vi "5.4-4.7.4-How Client.vi"() -> ()   [LabVIEW 2010]
doc: "This VI implements a client for the Named Service UDP Server.vi.\nIt connects to a service by specifying the server address and the name of the service. After sending a 'Hello' string to the server, the client receives the string sent by the server, displays the string and closes the connection.\n\n<b>Note:</b> This VI is built to work with the Named Service UDP Server.vi in UDP.llb."
uses:
  4-High Neurons/4.4-How Sensor Typedef.ctl
  4-High Neurons/4.0-Midbrain State.ctl
  4-High Neurons/4.0-Timing Badass.ctl
  <vilib>/Utility/tcp.llb/UDP Multicast Open.vi
  5.0-Global.vi
  5.7-UDP/5.7-UDP Check Checksum.vi
  <vilib>/addons/internet/NI_InternetTK_Common_VIs.lvlib
panel:
  out "Super Heart Beat":T1
  out "data":T2
  out "Error":errorcluster
  in  "stop":bool
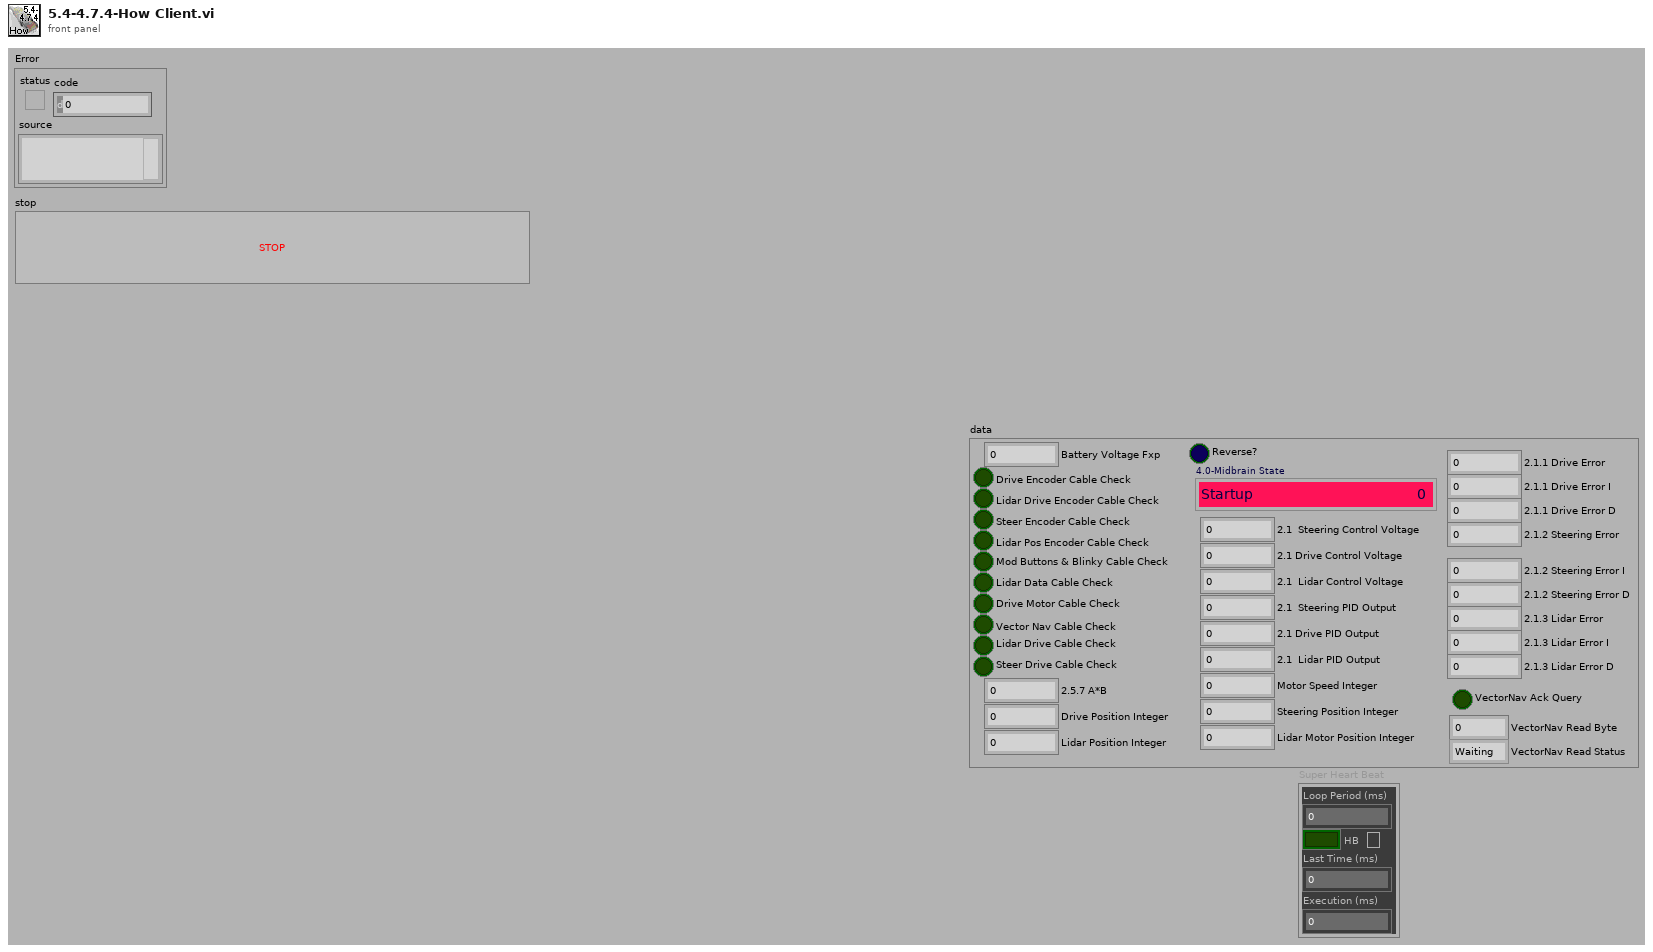
[diagram p1: front panel]
types:
  T1 = typedef "4.0-Timing Badass.ctl" = cluster{"Loop Period (ms)":u32, "HB":bool, "Last Time (ms)":u32, "Execution (ms)":u32}
  T2 = typedef "4.4-How Sensor Typedef.ctl" = cluster{"Motor Speed Integer":i32, "Drive Position Integer":i32, "Lidar Position Integer":i32, "Lidar Motor Position Integer":i32, "Steering Position Integer":i32, "Battery Voltage Fxp":dbl, "Drive Encoder Cable Check":bool, "Lidar Drive Encoder Cable Check":bool, "Steer Encoder Cable Check":bool, "Lidar Pos Encoder Cable Check":bool, "Mod Buttons & Blinky Cable Check":bool, "Lidar Data Cable Check":bool, "Drive Motor Cable Check":bool, "Vector Nav Cable Check":bool, "Lidar Drive Cable Check":bool, "Steer Drive Cable Check":bool, "Reverse?":bool, "2.1  Steering Control Voltage":dbl, "2.1 Drive Control Voltage":dbl, "2.1  Lidar Control Voltage":dbl, "2.5.7 A*B":dbl, "2.1  Steering PID Output":dbl, "2.1 Drive PID Output":dbl, "2.1  Lidar PID Output":dbl, "2.1.1 Drive Error":dbl, "2.1.1 Drive Error I":dbl, "2.1.1 Drive Error D":dbl, "2.1.2 Steering Error":dbl, "2.1.2 Steering Error I":dbl, "2.1.2 Steering Error D":dbl, "2.1.3 Lidar Error":dbl, "2.1.3 Lidar Error I":dbl, "2.1.3 Lidar Error D":dbl, "VectorNav Ack Query":bool, "VectorNav Read Byte":u8, "VectorNav Read Status":enum16{"Waiting", "Reading", "Done"}, "4.0-Midbrain State":T3}
  T3 = typedef "4.0-Midbrain State.ctl" = enum16{"Startup", "Waiting to Run", "Running-OlinOval", "Running-ChannelFollow", "Running-WallFollow", "Running-OpenTransit", "Running-Joystick Training", "Shutdown", "Restart"}
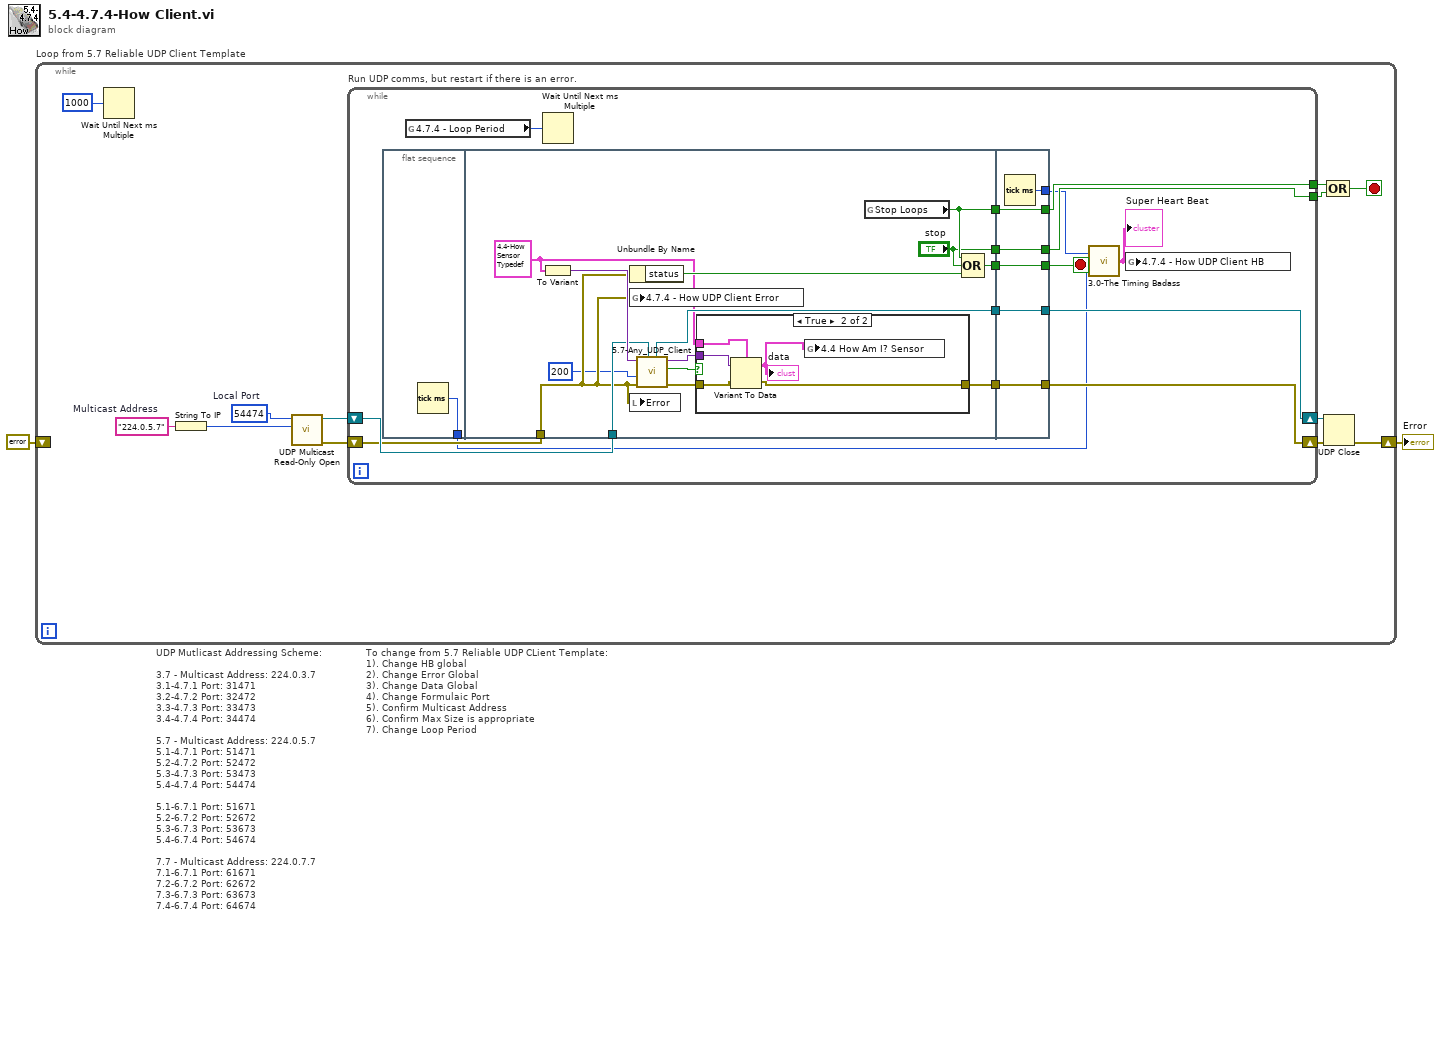
[diagram p0: block diagram]
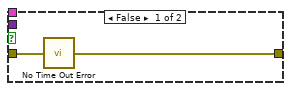
[diagram p2: hidden frame]
diagram:
  # "To change from 5.7 Reliable UDP CLient Template:\n1). Change HB global\n2). Change Error Global\n3). Change Data Global\n4). Change Formulaic Port\n5). Confirm Multicast Address\n6). Confirm Max Size is appropriate\n7). Change Loop Period"
  # "UDP Mutlicast Addressing Scheme:\n\n3.7 - Multicast Address: 224.0.3.7\n3.1-4.7.1 Port: 31471\n3.2-4.7.2 Port: 32472\n3.3-4.7.3 Port: 33473\n3.4-4.7.4 Port: 34474\n\n5.7 - Multicast Address: 224.0.5.7\n5.1-4.7.1 Port: 51471\n5.2-4.7.2 Port: 52472\n5.3-4.7.3 Port: 53473\n5.4-4.7.4 Port: 54474\n\n5.1-6.7.1 Port: 51671\n5.2-6.7.2 Port: 52672\n5.3-6.7.3 Port: 53673\n5.4-6.7.4 Port: 54674\n\n7.7 - Multicast Address: 224.0.7.7\n7.1-6.7.1 Port: 61671\n7.2-6.7.2 Port: 62672\n7.3-6.7.3 Port: 63673\n7.4-6.7.4 Port: 64674"
  n1 = while "Loop from 5.7 Reliable UDP Client Template" {
    shift-right: [w9] -> w2
    shift-left: errorcluster {"status"=FALSE, "code"=0, "source"=""} ("error out") -> [_]
    stop <- w12 stop-if-true
    w5 = u16 54474  # Local Port
    w7 = "224.0.5.7"  # Multicast Address
    n2 = Wait Until Next ms Multiple(millisecond multiple=u32 1000) -> ()  [unwired: 1 out]
    n3 = String To IP(1:w7) -> (0:w6:u32)
    n4 = call-poly <vilib>:"UDP Multicast Read-Only Open.vi"("multicast addr"=w6, "port"=w5) -> ("error out"=w3:errorcluster, "connection ID"=w4:refnum<k16>)  [unwired: 2 in, 6 out]
    n5 = while "Run UDP comms, but restart if there is an error." {
      tunnel: [w29] -> w14
      tunnel: [w28] -> w13
      shift-right: [w26] -> w11
      shift-left: w4 -> [w27]
      shift-right: [w25] -> w10
      shift-left: w3 -> [w24]
      stop <- w30 stop-if-true
      n6 = flat-sequence {
        tunnel: [w31] -> w16
        tunnel: w27 -> [w39]
        tunnel: w24 -> [w34]
        tunnel: [w45] -> w22
        tunnel: [w42] -> w21
        tunnel: ["stop"] -> w20
        tunnel: [w38] -> w19
        tunnel: [w37] -> w18
        tunnel: [w54] -> w25
        tunnel: [w55] -> w26
        tunnel: [w56] -> w28
        tunnel: [w57] -> w29
        tunnel: [w58] -> w30
        tunnel: w22 -> [w58]
        tunnel: w21 -> [w57]
        tunnel: w20 -> [w56]
        tunnel: w19 -> [w55]
        tunnel: w18 -> [w54]
        tunnel: [w53] -> w17
        frame #0 {
          n7 = Tick Count (ms)() -> (millisecond timer value=w31:u32)
        }
        frame #1 {
          w32 = T2 {"Motor Speed Integer"=0, "Drive Position Integer"=0, "Lidar Position Integer"=0, "Lidar Motor Position Integer"=0, "Steering Position Integer"=0, "Battery Voltage Fxp"=0.0, "Drive Encoder Cable Check"=FALSE, "Lidar Drive Encoder Cable Check"=FALSE, "Steer Encoder Cable Check"=FALSE, "Lidar Pos Encoder Cable Check"=FALSE, "Mod Buttons & Blinky Cable Check"=FALSE, "Lidar Data Cable Check"=FALSE, "Drive Motor Cable Check"=FALSE, "Vector Nav Cable Check"=FALSE, "Lidar Drive Cable Check"=FALSE, "Steer Drive Cable Check"=FALSE, "Reverse?"=FALSE, "2.1  Steering Control Voltage"=0.0, "2.1 Drive Control Voltage"=0.0, "2.1  Lidar Control Voltage"=0.0, "2.5.7 A*B"=0.0, "2.1  Steering PID Output"=0.0, "2.1 Drive PID Output"=0.0, "2.1  Lidar PID Output"=0.0, "2.1.1 Drive Error"=0.0, "2.1.1 Drive Error I"=0.0, "2.1.1 Drive Error D"=0.0, "2.1.2 Steering Error"=0.0, "2.1.2 Steering Error I"=0.0, "2.1.2 Steering Error D"=0.0, "2.1.3 Lidar Error"=0.0, "2.1.3 Lidar Error I"=0.0, "2.1.3 Lidar Error D"=0.0, "VectorNav Ack Query"=FALSE, "VectorNav Read Byte"=0, "VectorNav Read Status"=enum."Waiting", "4.0-Midbrain State"=enum."Startup"} ("4.4 How Am I? Sensor")
          n8 = To Variant(anything=w32) -> (Variant=w44:variant)
          n9 = Unbundle By Name(w34) -> ("status"=w40:bool)
          n10 = global write "5.0-Global.vi" "4.7.4 - How UDP Client Error"(w34) -> ()
          n11 = local write "Error"(w34) -> ()
          n12 = call "5.7-Any_UDP_Client.vi"("Port In"=w39, "error In"=w34, "Max Size"=200, "DataTypeIn"=w44) -> ("Error Out"=w36:errorcluster, "Check Passed"=w35:bool, "DataOut"=w43:variant, "Port out"=w38:refnum<k16>)  [unwired: 4 in]
          n13 = case "Ignore Timeouts" shown="True" w35 {
            tunnel: w43 -> [_ w52]
            tunnel: w32 -> [_ w51]
            tunnel: w36 -> [w47 w50]
            tunnel: [w46 w49] -> w37
            frame False {
              n14 = call <vilib>:"No Time Out Error.vi"("error in (no error)"=w47) -> ("error out"=w46:errorcluster)  [unwired: 14 in]
            }
            frame True {
              n15 = Variant To Data(error in=w50, Variant=w52, type=w51) -> (error out=w49:errorcluster, data=w48:T2)
              "data" <- w48
              n16 = global write "5.0-Global.vi" "4.4 How Am I? Sensor"(w48) -> ()
            }
          }
          n17 = global read "5.0-Global.vi" "Stop Loops"() -> (w42:bool)
          n18 = Compound Arithmetic op=OR(w42, "stop", w40) -> (w45:bool)
        }
        frame #2 {
          n19 = Tick Count (ms)() -> (millisecond timer value=w53:u32)
        }
      }
      n20 = global read "5.0-Global.vi" "4.7.4 - Loop Period"() -> (w23:u32)
      n21 = Wait Until Next ms Multiple(millisecond multiple=w23) -> ()  [unwired: 1 out]
      n22 = call "3.0-The Timing Badass.vi"("Start"=w16, "End"=w17) -> ("Super Heart Beat"=w15:T1)
      "Super Heart Beat" <- w15
      n23 = global write "5.0-Global.vi" "4.7.4 - How UDP Client HB"(w15) -> ()
    }
    n24 = UDP Close(connection ID=w11, 8:w10) -> (error out=w9:errorcluster)  [unwired: 1 out]
    n25 = Compound Arithmetic op=OR(w14, w13) -> (w12:bool)
  }
  "Error" <- w2
